vi "LoadColorSpace.vi"(11 "relative path":string) -> (2 "white":cluster{dbl[], dbl[]}, 3 "gamut":cluster{dbl[], dbl[]})   [LabVIEW 2011]
uses:
  <vilib>/Utility/file.llb/Read From Spreadsheet File (DBL).vi
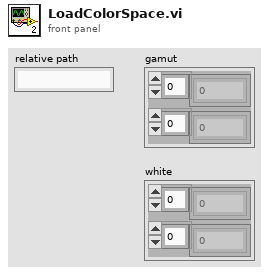
[diagram p1: front panel]
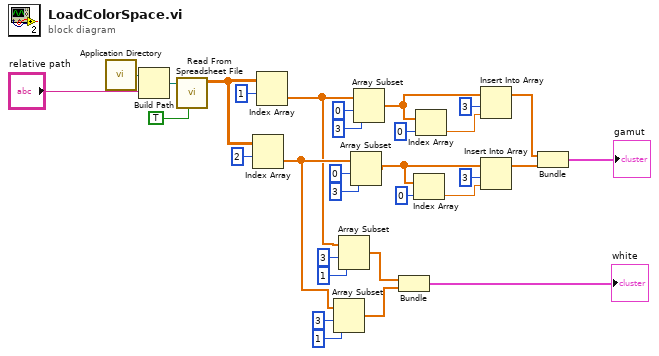
[diagram p0: block diagram]
diagram:
  n1 = call <vilib>:"Application Directory.vi"() -> ("Application Directory"=w1:path)
  n2 = Build Path(base path=w1, name or relative path="relative path") -> (appended path=w2:path)
  n3 = call-poly <vilib>:"Read From Spreadsheet File.vi"("transpose (no:F)"=TRUE, "file path (dialog if empty)"=w2) -> ("all rows"=w6:dbl[][])  [unwired: 5 in, 4 out]
  n4 = Index Array(array=w6, index (row)=2) -> (element=w22:dbl[])  [unwired: 1 in]
  n5 = Index Array(array=w6, index (row)=1) -> (element=w17:dbl[])  [unwired: 1 in]
  n6 = Array Subset(array=w22, index=3, length=1) -> (w16:dbl[])
  n7 = Array Subset(array=w17, index=3, length=1) -> (w15:dbl[])
  n8 = Array Subset(array=w22, index=0, length=3) -> (w23:dbl[])
  n9 = Array Subset(array=w17, index=0, length=3) -> (w29:dbl[])
  n10 = Bundle(w15, w16) -> (→"white":cluster{dbl[], dbl[]})  [unwired: 1 in]
  n11 = Index Array(array=w23, index=0) -> (element=w25:dbl)
  n12 = Index Array(array=w29, index=0) -> (element=w28:dbl)
  n13 = Insert Into Array(array=w29, index=3, new element=w28) -> (w30:dbl[])
  n14 = Insert Into Array(array=w23, index=3, new element=w25) -> (w31:dbl[])
  n15 = Bundle(w30, w31) -> (→"gamut":cluster{dbl[], dbl[]})  [unwired: 1 in]
